vi "GetFreeLabel.vi"(6 "error in":errorcluster, 9 "Decoration in":refnum<class "Decoration.lvclass">) -> (0 "error out":errorcluster, 3 "Decoration out":refnum<class "Decoration.lvclass">, 4 "Items":T1[](array[typedef]))   [LabVIEW 2014, in "Raspberry Pi Compatible Compiler for LabVIEW.lvlib" / "PythonConverter_GUI.lvclass"]
uses:
  PythonConverter_GUI.lvclass
  VI Interpreter/Classes/Decoration/Decoration.lvclass
  PythonConfiguration/TypeDefs/ItemTD.ctl
  VI Interpreter/Classes/Text/Text.lvclass/Text.ctl
  VI Interpreter/Classes/Decoration/Decoration.lvclass/Decoration.ctl
  VI Interpreter/Classes/Text/Text.lvclass
  PythonConfiguration/PythonConfiguration.lvclass
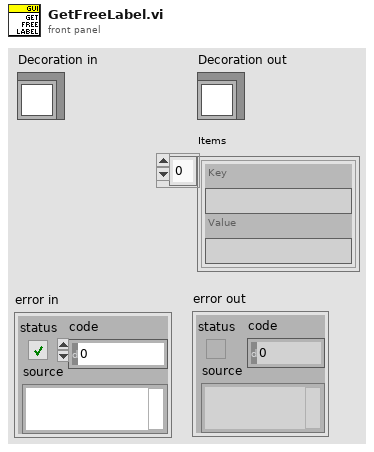
[diagram p1: front panel]
types:
  T1 = typedef "Raspberry Pi Compatible Compiler for LabVIEW.lvlib/PythonConfiguration.lvclass/ItemTD.ctl" = cluster{"Key":string, "Value":string}
  T2 = typedef "LVFontTypeDef.ctl" = cluster{"Font Name":string, "Size":u16, "Bold":bool, "Italic":bool, "Underline":bool, "Strikeout":bool, "Color":u32}
  T3 = typedef "LVBoundsTypeDef.ctl" = cluster{"Width":u32, "Height":u32}
  T4 = typedef "LVPositionTypeDef.ctl" = cluster{"Left":i32, "Top":i32}
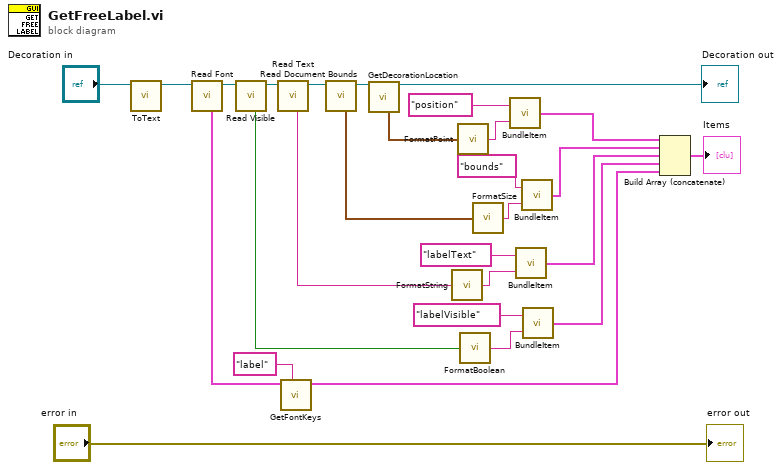
[diagram p0: block diagram]
diagram:
  n1 = call "ToText.vi"("Generic"="Decoration in") -> ("Text out"=w5:refnum<class "Text.lvclass">)  [unwired: 9 in, 1 out]
  n2 = call "Read Font.vi"("Text in"=w5) -> ("Text out"=w15:refnum<class "Text.lvclass">, "Font"=w14:T2)  [unwired: 7 in]
  n3 = call "Read Visible.vi"("Decoration in"=w15) -> ("Decoration out"=w20:refnum<class "Text.lvclass">, "Visible"=w16:bool)  [unwired: 7 in]
  n4 = call "Read Text.vi"("Text in"=w20) -> ("Text out"=w4:refnum<class "Text.lvclass">, "Text"=w25:string)  [unwired: 7 in]
  n5 = call "GetFontKeys.vi"("name"="label", "Font"=w14) -> ("font items"=w12:T1[])  [unwired: 7 in]
  n6 = call "Read Document Bounds.vi"("Text in"=w4) -> ("Text out"=w3:refnum<class "Text.lvclass">, "Document Bounds"=w11:T3)  [unwired: 7 in]
  n7 = call "GetDecorationLocation.vi"("Decoration in"=w3) -> ("Decoration out"=→"Decoration out":refnum<class "Text.lvclass">, "Position"=w1:T4)  [unwired: 6 in, 1 out]
  n8 = call "FormatString.vi"("String"=w25) -> ("value"=w24:string)  [unwired: 1 in]
  n9 = call "FormatPoint.vi"("point"=w1) -> ("value"=w27:string)
  n10 = call "FormatBoolean.vi"("boolean"=w16) -> ("value"=w17:string)
  n11 = call "FormatSize.vi"("size"=w11) -> ("value"=w9:string)
  n12 = call "BundleItem.vi"("Value"=w27, "Key"="position") -> ("Item"=w10:T1)
  n13 = call "BundleItem.vi"("Value"=w24, "Key"="labelText") -> ("Item"=w22:T1)
  n14 = call "BundleItem.vi"("Value"=w9, "Key"="bounds") -> ("Item"=w8:T1)
  n15 = call "BundleItem.vi"("Value"=w17, "Key"="labelVisible") -> ("Item"=w18:T1)
  n16 = Build Array (concatenate)(w10, w8, w22, w18, w12) -> (→"Items":T1[])
  "error out" <- "error in"
